vi "Simple_Power_Meter_Read.vi"(7 "Config String":string, 8 "error in (no error)":errorcluster, 9 "Expected Power(dBm)":dbl, 10 "Sample_count":u64 max=1024, 11 "VISA resource name":refnum<visa-resource-name>) -> (0 "error out":errorcluster, 2 "Measurement":dbl)   [LabVIEW 2025, in "Interface Functions.lvlib"]
uses:
  Interface Functions.lvlib
  <instrlib>/Agilent U2000 Series/Agilent U2000 Series.lvlib
panel:
  out "output array":string[](array[string])
  out "read buffer 2":string
  out "read buffer":string
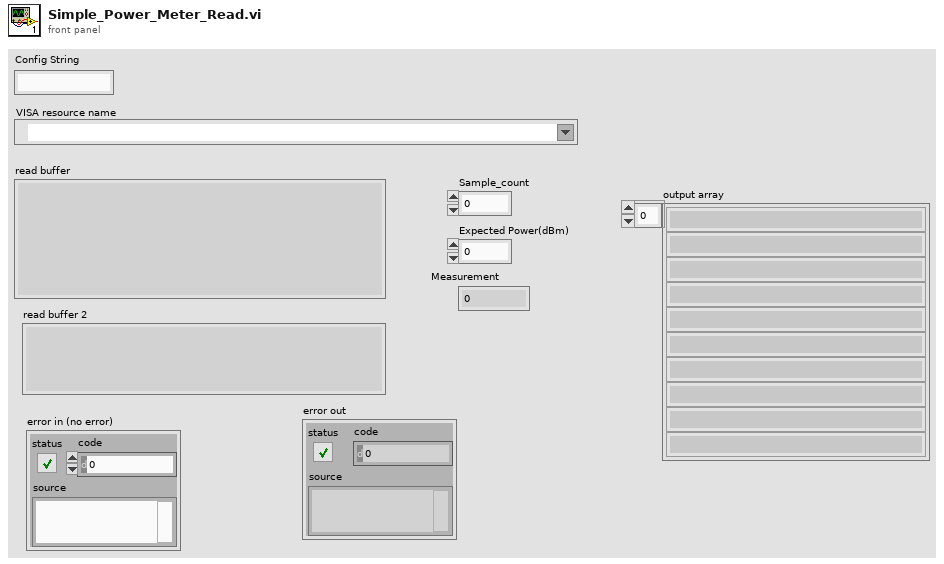
[diagram p1: front panel]
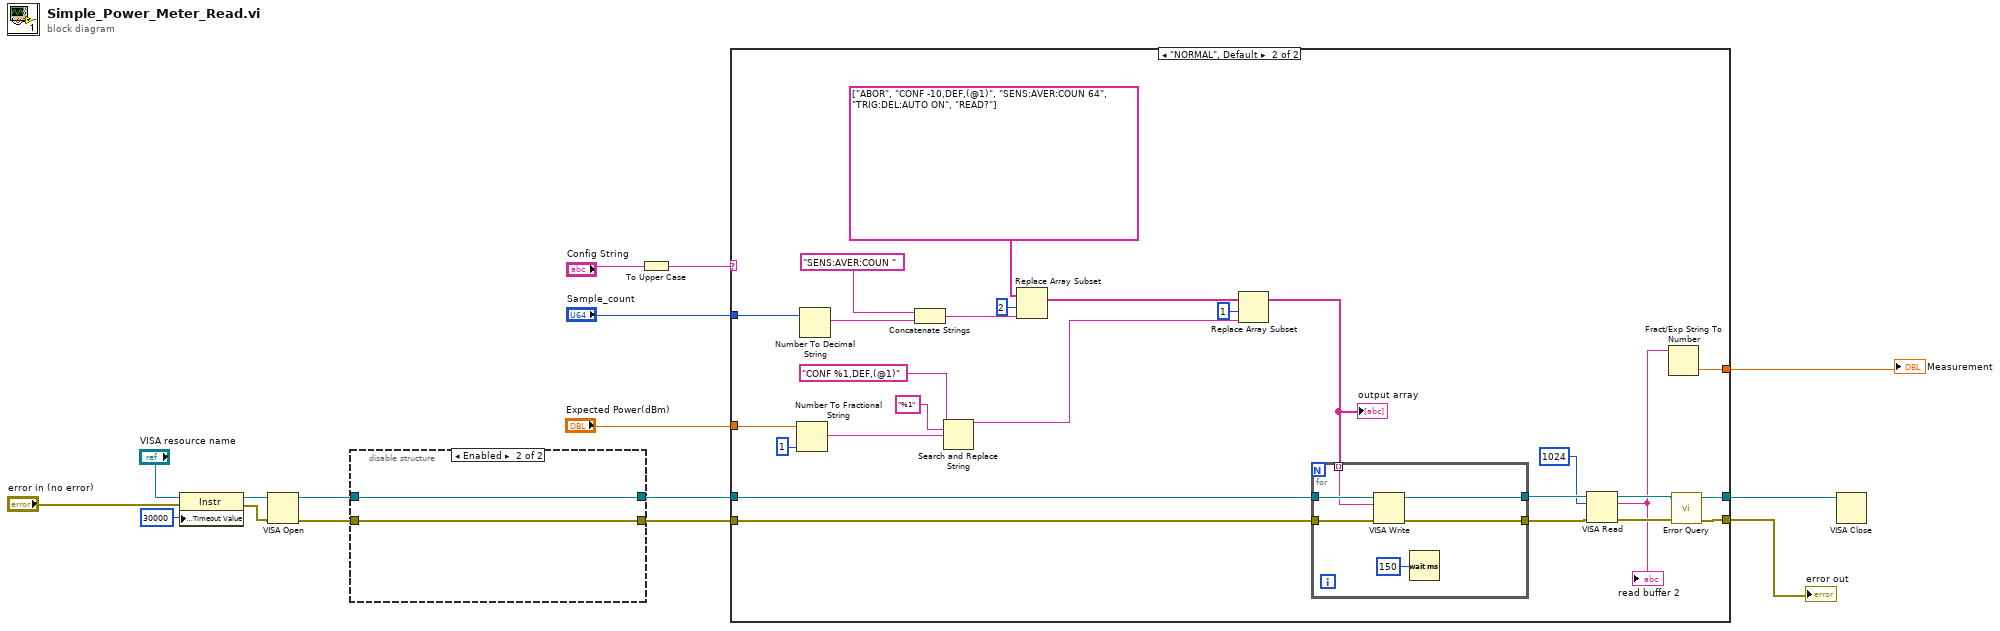
[diagram p0: block diagram]
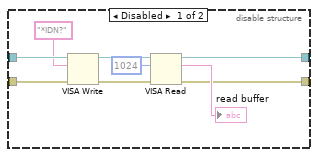
[diagram p2: hidden frame]
diagram:
  n1 = property class="Instr"(reference="VISA resource name", error in="error in (no error)", "General Settings:Timeout Value"=u32 30000) -> (reference out=w14:refnum<visa-resource-name>, error out=w5:errorcluster)
  n2 = VISA Open(error in (no error)=w5, VISA resource name=w14) -> (VISA resource name=w16:refnum<visa-resource-name>, error out=w7:errorcluster)  [unwired: 3 in]
  n3 = disable-structure shown="Enabled" {
    disable-tunnel: w16 -> [w25 w27]
    disable-tunnel: [w20 w27] -> w9
    disable-tunnel: w7 -> [w19 w26]
    disable-tunnel: [w17 w26] -> w6
    frame Disabled {
      n4 = VISA Write(VISA resource name=w25, write buffer="*IDN?", error in (no error)=w19) -> (VISA resource name out=w23:refnum<visa-resource-name>, error out=w18:errorcluster)  [unwired: 1 out]
      n5 = VISA Read(VISA resource name=w23, byte count=u32 1024, error in (no error)=w18) -> (VISA resource name out=w20:refnum<visa-resource-name>, read buffer=→"read buffer":string, error out=w17:errorcluster)  [unwired: 1 out]
    }
    frame Enabled {
    }
  }
  n6 = To Upper Case(1:"Config String") -> (0:w1:string)
  n7 = case shown="\"NORMAL\", Default" w1 {
    tunnel: "Sample_count" -> [_ w54]
    tunnel: "Expected Power(dBm)" -> [_ w49]
    tunnel: w9 -> [w29 w38]
    tunnel: [w29 w35] -> w8
    tunnel: w6 -> [w28 w37]
    tunnel: [w28 w34] -> w4
    tunnel: [_ w31] -> w2
    frame "BURST" {
    }
    frame "NORMAL", Default {
      n8 = Number To Fractional String(number=w49, precision (6)=i16 1) -> (F-format string=w43:string)  [unwired: 2 in]
      n9 = Number To Decimal String(number=w54) -> (decimal integer string=w52:string)  [unwired: 1 in]
      n10 = Concatenate Strings("SENS:AVER:COUN ", w52) -> (w51:string)
      n11 = Search and Replace String(input string="CONF %1,DEF,(@1)", search string="%1", replace string=w43) -> (result string=w42:string)  [unwired: 5 in, 3 out]
      n12 = Replace Array Subset(array=string[] ["ABOR", "CONF -10,DEF,(@1)", "SENS:AVER:COUN 64", "TRIG:DEL:AUTO ON", "READ?"], new element=w51, index=2) -> (w47:string[])
      n13 = Replace Array Subset(array=w47, new element=w42, index=1) -> (w39:string[])
      "output array" <- w39
      n14 = for {
        tunnel: w39 -> [w58] mode=indexing
        tunnel: w38 -> [w61]
        tunnel: [w60] -> w41
        tunnel: w37 -> [w57]
        tunnel: [w56] -> w36
        n15 = VISA Write(VISA resource name=w61, write buffer=w58, error in (no error)=w57) -> (VISA resource name out=w60:refnum<visa-resource-name>, error out=w56:errorcluster)  [unwired: 1 out]
        n16 = Wait (ms)(milliseconds to wait=u32 150) -> ()  [unwired: 1 out]
      }
      n17 = VISA Read(VISA resource name=w41, byte count=u32 1024, error in (no error)=w36) -> (VISA resource name out=w33:refnum<visa-resource-name>, read buffer=w30:string, error out=w32:errorcluster)  [unwired: 1 out]
      "read buffer 2" <- w30
      n18 = Fract/Exp String To Number(string=w30) -> (number=w31:dbl)  [unwired: 3 in, 1 out]
      n19 = call <instrlib>:"Error Query.vi"("error in (no error)"=w32, "VISA resource name"=w33) -> ("error out"=w34:errorcluster, "VISA resource name out"=w35:refnum<visa-resource-name>)  [unwired: 8 out]
    }
  }
  "error out" <- w4
  "Measurement" <- w2
  n20 = VISA Close(VISA resource name=w8) -> ()  [unwired: 1 in, 1 out]
